vi "templates switch template style.vi"(6 "User":string, 7 "POST Parameters":T1, 8 "error in (no error)":errorcluster, 9 "Keys in":T1, 10 "sxTemplateId":string, 11 "Connection Refnum In":T2) -> (0 "error out":errorcluster, 1 "HTM Keys out":T1, 2 "sEditor":string, 3 "Connection Refnum Out":T2)   [LabVIEW 2011]
uses:
  Addons/internet/utils/keyedarr.llb/Keyed Array.ctl
  SI.LIB/ODBC/SQL Controls/Connection Refnum.ctl
  Addons/internet/utils/strutil.llb/Case Matching.ctl
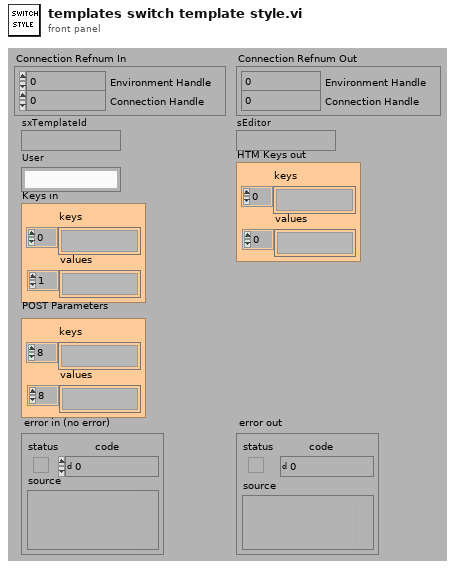
[diagram p1: front panel]
types:
  T1 = typedef "Keyed Array.ctl" = cluster{"keys":string[], "values":string[]}
  T2 = typedef "Connection Refnum.ctl" = cluster{"Environment Handle":i32, "Connection Handle":i32}
  T3 = typedef "Case Matching.ctl" = enum16{"a != A", "a == A", "system"}
  T4 = typedef "Template Record.ctl" = cluster{"ixTemplate":i32, "sxTemplateId":string, "sDescription":string, "sCreator":string, "tCreationDate":timestamp, "sModifier":string, "tModifiedDate":timestamp, "sType":string, "sStyle":string, "sFormat":string, "dWidth":dbl, "dHeight":dbl, "sFilename":string, "sScript":string, "sLayout":string, "sEditor":string, "sStyleProcess":string}
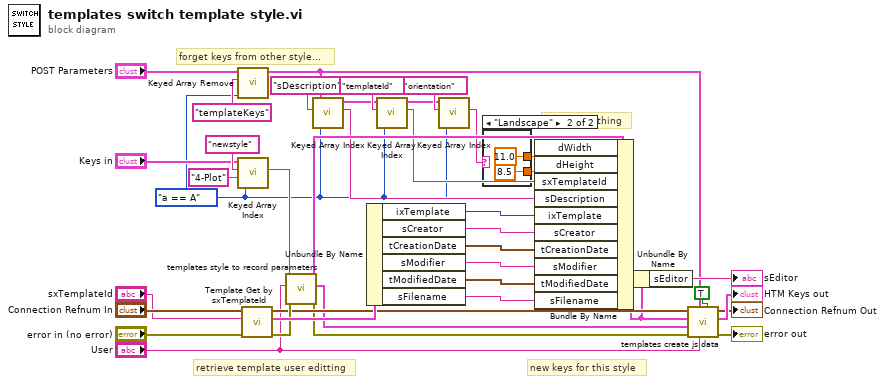
[diagram p0: block diagram]
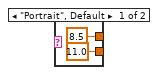
[diagram p2: hidden frame]
diagram:
  w4 = Case_Matching."a == A" ("case matching (sensitive)")
  # "forget keys from other style..."
  # "new keys for this style"
  # "swap everything"
  # "retrieve template user editting"
  n1 = call "Keyed Array Remove.vi"("case matching (sensitive)"=w4, "key"="templateKeys", "array in"="POST Parameters") -> ("array out"=w7:T1)  [unwired: 4 out]
  n2 = call "Keyed Array Index.vi"("case matching (sensitive)"=w4, "default value"="4-Plot" ("key"), "key"="newstyle", "array in"="Keys in") -> ("value"=w10:string)  [unwired: 3 out]
  n3 = call "Template Get by sxTemplateId.vi"("error in (no error)"="error in (no error)", "sxTemplateId (\"\")"="sxTemplateId", "Connection Refnum"="Connection Refnum In") -> ("error out"=w24:errorcluster, "Template Record"=w30:T4, "Connection Refnum"=w22:T2)  [unwired: 6 out]
  n4 = call "templates style to record parameters.vi"("error in (no error)"=w24, "user"="User", "template style"=w10) -> ("error out"=w21:errorcluster, "Parameters"=w19:T1, "Template Record"=w23:T4)  [unwired: 6 out]
  n5 = call "Keyed Array Index.vi"("case matching (sensitive)"=w4, "key"="sDescription", "array in"=w7) -> ("value"=w8:string, "duplicate array"=w12:T1)  [unwired: 1 in, 2 out]
  n6 = Unbundle By Name(w30) -> ("ixTemplate"=w11:i32, "sCreator"=w29:string, "tCreationDate"=w28:timestamp, "sModifier"=w27:string, "tModifiedDate"=w26:timestamp, "sFilename"=w25:string)
  n7 = call "Keyed Array Index.vi"("case matching (sensitive)"=w4, "key"="templateId", "array in"=w12) -> ("value"=w9:string, "duplicate array"=w5:T1)  [unwired: 1 in, 2 out]
  n8 = call "Keyed Array Index.vi"("case matching (sensitive)"=w4, "key"="orientation", "array in"=w5) -> ("value"=w3:string)  [unwired: 1 in, 3 out]
  n9 = case shown="\"Landscape\"" w3 {
    tunnel: [8.5 ("dWidth") 11.0 ("dWidth")] -> w1
    tunnel: [11.0 ("dWidth") 8.5 ("dWidth")] -> w2
    frame "Portrait", Default {
    }
    frame "Landscape" {
    }
  }
  n10 = Bundle By Name(cluster=w23, "dWidth"=w1, "dHeight"=w2, "sxTemplateId"=w9, "sDescription"=w8, "ixTemplate"=w11, "sCreator"=w29, "tCreationDate"=w28, "sModifier"=w27, "tModifiedDate"=w26, "sFilename"=w25) -> (w20:T4)
  n11 = Unbundle By Name(w20) -> ("sEditor"=→"sEditor":string)
  n12 = call "templates create js data.vi"("Changes?"=TRUE, "sxUsername"="User", "POST Parameters"=w7, "error in (no error)"=w21, "template Parameters"=w19, "Template Record"=w20, "Connection Refnum"=w22) -> ("error out"=→"error out":errorcluster, "HTM Keys"=→"HTM Keys out":T1, "Connection Refnum"=→"Connection Refnum Out":T2)  [unwired: 2 out]
